vi "Read Parameters (array).vi"(8 "error in (no error)":errorcluster, 11 "Run Instance in":refnum<class "Run Instance.lvclass">) -> (0 "error out":errorcluster, 2 "Parameters":string[][](array[string]), 3 "Run Instance out":refnum<class "Run Instance.lvclass">)   [LabVIEW 2020, in "TALOS.lvlib" / "Run Utilities.lvlib" / "Run Instance.lvclass"]
uses:
  Run Instance.lvclass
  Run Instance.lvclass/Run Instance.ctl
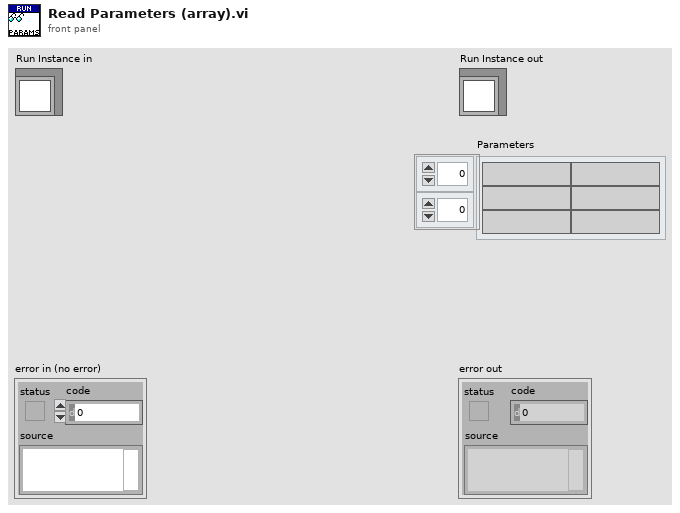
[diagram p1: front panel]
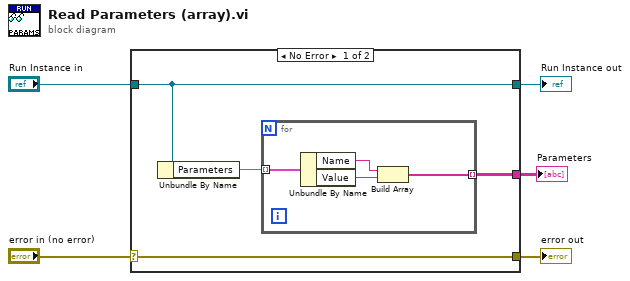
[diagram p0: block diagram]
diagram:
  n1 = case shown="No Error" "error in (no error)" {
    selector: "error in (no error)" -> [w9 w14]
    tunnel: [w9 w14] -> w4
    tunnel: [w8 w15] -> w2
    tunnel: "Run Instance in" -> [w8 w15]
    tunnel: [w6 _] -> w1
    frame No Error {
      n2 = Unbundle By Name(w8) -> ("Parameters"=w7:map{string, string})
      n3 = for {
        tunnel: w7 -> [w13] mode=indexing
        tunnel: [w10] -> w6 mode=indexing
        n4 = Unbundle By Name(w13) -> ("Name"=w12:string, "Value"=w11:string)
        n5 = Build Array(w12, w11) -> (w10:string[])
      }
    }
    frame Error {
    }
  }
  "error out" <- w4
  "Run Instance out" <- w2
  "Parameters" <- w1
